vi "4155C Config VMU.vi"(0 "VISA session":refnum<visa-resource-name>, 2 "Range mode":u16(ring) items=["Auto", "Limited", "Fixed"], 5 "unit to configure":u32(slide) max=1, 11 "error in (no error)":errorcluster, 12 "V name (max 6 chars)":string) -> (4 "dup VISA resource name":refnum<visa-resource-name>, 15 "error out":errorcluster)   [LabVIEW 2009]
doc: "This VI configures an VMU for SWEEP mode measurement."
panel:
  in  "Measurement Range":u32(slide) max=2
  in  "Discharge on/off":bool
  in  "Measurement mode":u32(slide) max=1
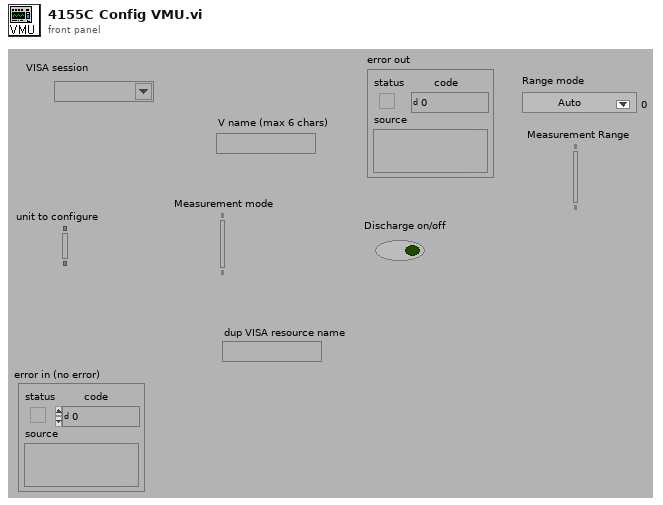
[diagram p1: front panel]
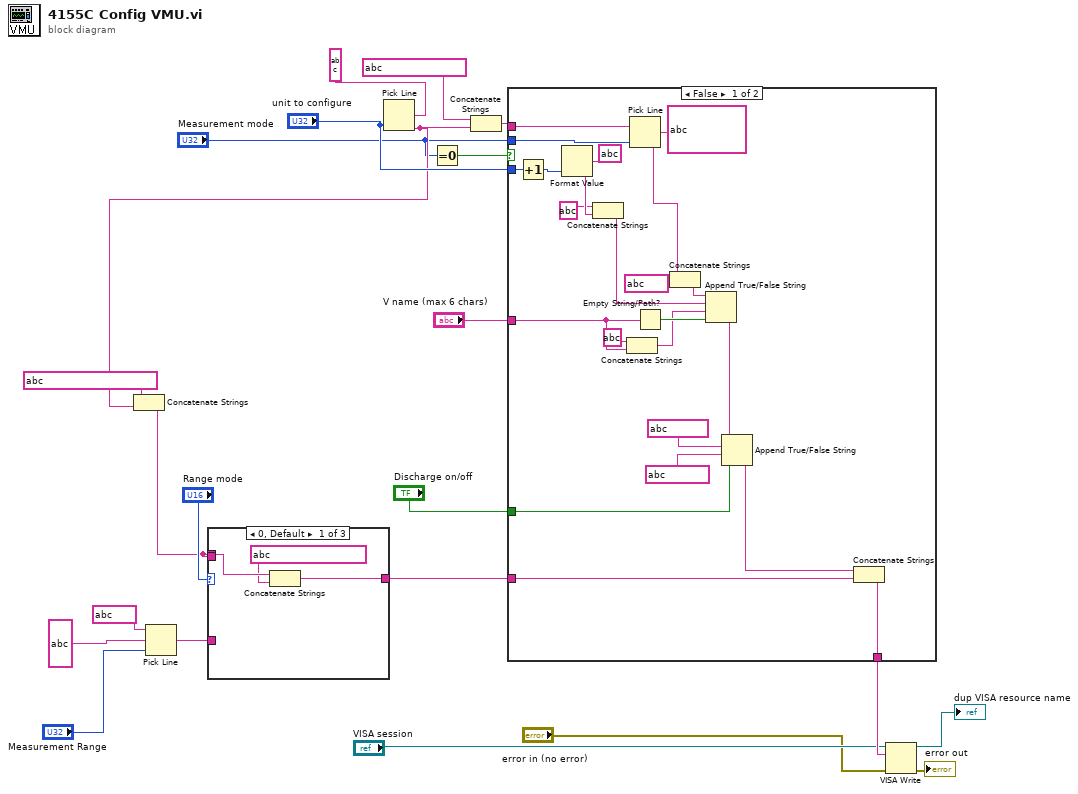
[diagram p0: block diagram]
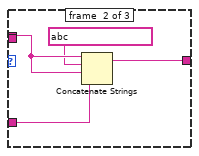
[diagram p2: hidden frame]
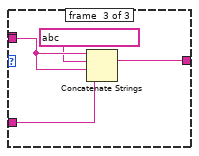
[diagram p3: hidden frame]
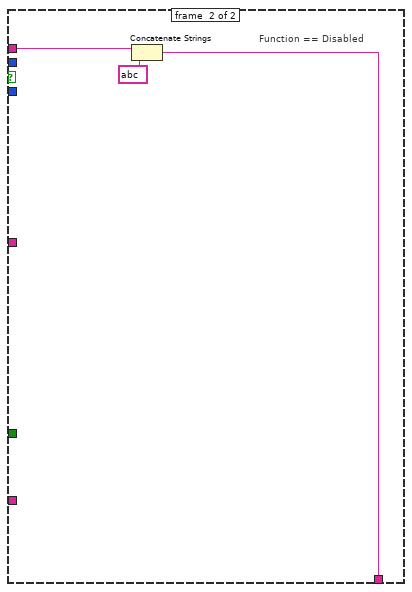
[diagram p4: hidden frame]
diagram:
  n1 = Pick Line(string ("")=string ?, multi-line string=string ?, line index="Measurement Range") -> (output string=w10:string)
  n2 = Pick Line(multi-line string=string ?, line index="unit to configure") -> (output string=w7:string)  [unwired: 1 in]
  n3 = Concatenate Strings(string ? ("Substring"), w7) -> (w5:string)
  n4 = case shown="0, Default" "Range mode" {
    tunnel: w10 -> [_ w29 w31]
    tunnel: [w23 w26 w32] -> w9
    tunnel: w5 -> [w25 w28 _]
    tunnel: w5 -> [_ _ w33]
    frame #0 {
      n5 = Concatenate Strings(w25, string ? ("multi-line string")) -> (w23:string)
    }
    frame #1 {
      n6 = Concatenate Strings(w28, string ? ("multi-line string"), w28, w29) -> (w26:string)
    }
    frame #2 {
      n7 = Concatenate Strings(w33, string ? ("multi-line string"), w33, w31) -> (w32:string)
    }
  }
  n8 = Equal To 0?(x="Measurement mode") -> (x = 0?=w18:bool)
  n9 = Concatenate Strings(string ?, w7) -> (w12:string)
  n10 = case shown="False" w18 {
    tunnel: w12 -> [w38 w59]
    tunnel: "Measurement mode" -> [w55 _]
    tunnel: "unit to configure" -> [w42 _]
    tunnel: "V name (max 6 chars)" -> [w46 _]
    tunnel: "Discharge on/off" -> [w41 _]
    tunnel: [w39 w57] -> w20
    tunnel: w9 -> [w37 _]
    frame #0 {
      n11 = Increment(x=w42) -> (x+1=w35:u32)
      n12 = Format Value(format string=string ?, value (0)=w35) -> (output string=w53:string)  [unwired: 1 in]
      n13 = Concatenate Strings(string ?, w53) -> (w49:string)
      n14 = Concatenate Strings(string ?, w46) -> (w45:string)
      n15 = Pick Line(string ("")=w38, multi-line string=string ?, line index=w55) -> (output string=w36:string)
      n16 = Empty String/Path?(string/path=w46) -> (empty?=w48:bool)
      n17 = Concatenate Strings(w36, string ?) -> (w50:string)
      n18 = Append True/False String(1:w48, 2:w45, 3:w49, 4:w50) -> (0:w34:string)
      n19 = Append True/False String(1:w41, 2:string ?, 3:string ?, 4:w34) -> (0:w40:string)
      n20 = Concatenate Strings(w40, w37) -> (w39:string)
    }
    frame #1 {
      # "Function == Disabled"
      n21 = Concatenate Strings(w59, string ?) -> (w57:string)
    }
  }
  n22 = VISA Write(VISA resource name="VISA session", write buffer=w20, error in (no error)="error in (no error)") -> (VISA resource name out=→"dup VISA resource name":refnum<visa-resource-name>, error out=→"error out":errorcluster)  [unwired: 1 out]
